vi "Read_Start_Key.vi"(8 "error in (no error)":errorcluster caption="错误输入（无错误）") -> (0 "error out":errorcluster caption="错误输出", 1 "子字符串":string, 2 "子字符串之后":string, 3 "读取缓冲区":string)   [LabVIEW 2018]
uses:
  Global.vi
  <vilib>/Instr/_visa.llb/VISA Configure Serial Port (Instr).vi
panel:
  out "RS232_1":refnum<visa-resource-name>
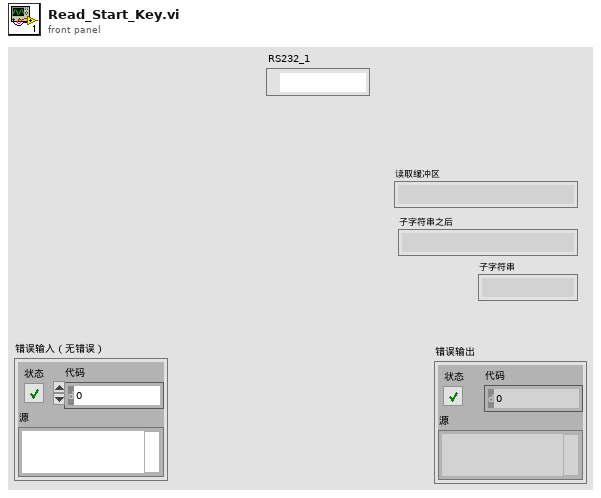
[diagram p1: front panel]
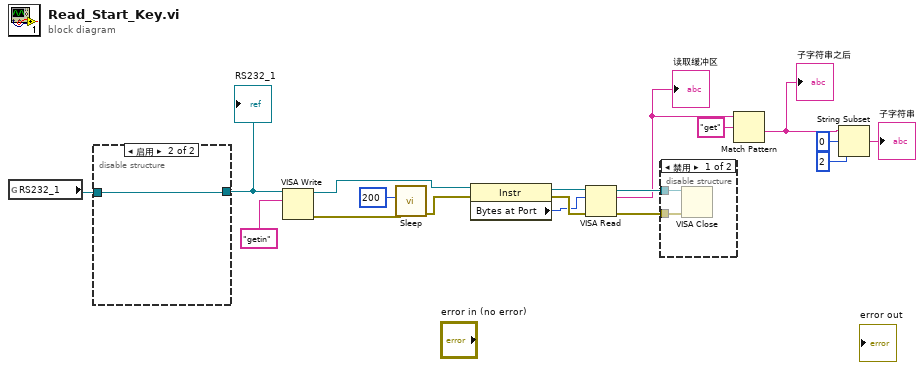
[diagram p0: block diagram]
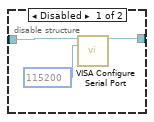
[diagram p3: hidden frame]
diagram:
  n1 = global read "Global.vi" "RS232_1"() -> (w10:refnum<visa-resource-name>)
  n2 = disable-structure shown="启用" {
    disable-tunnel: w10 -> [w21 w22]
    disable-tunnel: [w20 w22] -> w9
    frame Disabled {
      n3 = call-poly "VISA Configure Serial Port"("VISA resource name"=w21, "baud rate (9600)"=u32 115200) -> ("VISA resource name out"=w20:refnum<visa-resource-name>)  [unwired: 12 in, 1 out]
    }
    frame Enabled {
    }
  }
  "RS232_1" <- w9
  n4 = VISA Write(VISA resource name=w9, write buffer="getin" ("写入缓冲区")) -> (VISA resource name out=w15:refnum<visa-resource-name>, error out=w16:errorcluster)  [unwired: 1 in, 1 out]
  n5 = call "Sleep.vi"("error in (no error)"=w16, "等待时间（毫秒）"=u32 200) -> ("error out"=w14:errorcluster)  [unwired: 9 in]
  n6 = property class="Instr"(reference=w15, error in=w14) -> (reference out=w13:refnum<visa-resource-name>, error out=w12:errorcluster, "Bytes at Port"=w11:u32)
  n7 = VISA Read(VISA resource name=w13, byte count=w11, error in (no error)=w12) -> (VISA resource name out=w8:refnum<visa-resource-name>, read buffer=w6:string, error out=w7:errorcluster)  [unwired: 1 out]
  "读取缓冲区" <- w6
  n8 = disable-structure shown="禁用" {
    disable-tunnel: w8 -> [w24 _]
    disable-tunnel: w7 -> [w23 _]
    frame Disabled {
      n9 = VISA Close(VISA resource name=w24, error in (no error)=w23) -> ()  [unwired: 1 out]
    }
    frame Enabled {
    }
  }
  n10 = Match Pattern(string=w6, regular expression="get" ("正则表达式")) -> (after substring=w4:string)  [unwired: 1 in, 3 out]
  "子字符串之后" <- w4
  n11 = String Subset(string=w4, offset (0)=0 ("偏移量(0)"), length (rest)=2 ("长度（剩余）")) -> (substring=→"子字符串":string)
